vi "WS1021 demo GUI.vi"(6 "Error Limits file":path, 7 "VNA ports":bool[](array[boolean])=[TRUE, FALSE, FALSE, FALSE], 8 "Error In":errorcluster, 9 "De-embedding files":path[](array[path]), 10 "Toggle 8.lvclass":refnum<class "Toggle 8.lvclass">, 11 "Vector Network Analyzer.lvclass":refnum<class "Vector Network Analyzer.lvclass">) -> (0 "Error Out":errorcluster, 2 "Toggle 8.lvclass 2":refnum<class "Toggle 8.lvclass">, 3 "Vector Network Analyzer.lvclass 2":refnum<class "Vector Network Analyzer.lvclass">)   [LabVIEW 2020]
uses:
  Instruments/Vector Network Analyzer/Vector Network Analyzer.lvclass
  Devices/Toggle 8/Toggle 8.lvclass
  WS1021 demo GUI settings.ctl
  <vilib>/addons/HF Network Analysis/Support VIs/Read SnP File (SnP).vi
  <vilib>/addons/HF Network Analysis/NI_HFNetworkAnalysis.lvlib
  Devices/PIC-device/PIC-Device.lvclass
panel:
  out "Error limits":cluster{"Array":i32[], "Array":dbl[]}
  out "ErrorvsOTP":cluster{i32[], dbl[]}[](graph) caption="Capacitance error vs Setting"
  out "Heading":string[](array[string])=["Frequency (MHz)", "Capacitance (pF)", "Resistance (Ohm)", "Q", "Cshunt1 (pF)", "Cshunt2 (pF)", "SRF (MHz)"]
  out "Capacitance (pF) at f1":dbl caption="Capacitance (pF)\n at 900MHz" format="%#.2g"
  in  "Mode":enum32{"Automatic mode", "Manual mode"}(radio)
  in  "OTP":i32(slide)=1 caption="Capacitance setting" min=1 max=64 step=1 scale=1.0..64.0
  in  "Settings UI":bool
  in  "Pause Button":bool
  in  "Exit Button":bool
  out "Status bar":string
  out "Time":string
  in  "CvsOTP":cluster{"OTP":i32[], "Capa":dbl[]}
  out "Q at f2":dbl caption="Q-Value \nat 2000MHz" format="%#.1g"
  out "CvsOTP Graph":cluster{i32[], dbl[]}[](graph) caption="Capacitance vs Setting"
  in  "Demo Mode":enum32{"Live mode", "Virtual mode"}(radio)
  out "Capa Graph":cluster{dbl[], dbl[]}(graph) caption="Capacitance vs Frequency"
  out "Q Graph":cluster{dbl[], dbl[]}(graph) caption="Q vs Frequency"
  in  "Settings":T1={"Specification"={"States"=32, "Cmin"=250.0, "Cmax"=2600.0}, "Extraction frequencies"={"Frequency for C (MHz)"=900.0, "Frequency for Q (MHz)"=2000.0, "Frequency, C_DC (MHz)"=100.0}, "Timeout (ms)"=250, "Model"=enum."pi", "Topology"=enum."Series", "Error limits"=path ""}
  out "Status text box":string
  out "Data":dbl[][](array[numeric]) caption="Frequency,C, R, Q, L, Cshunt1/2, Rshunt1/2, Lshunt1/2, SRF"
  # "Digitally Tunable Capacitor"
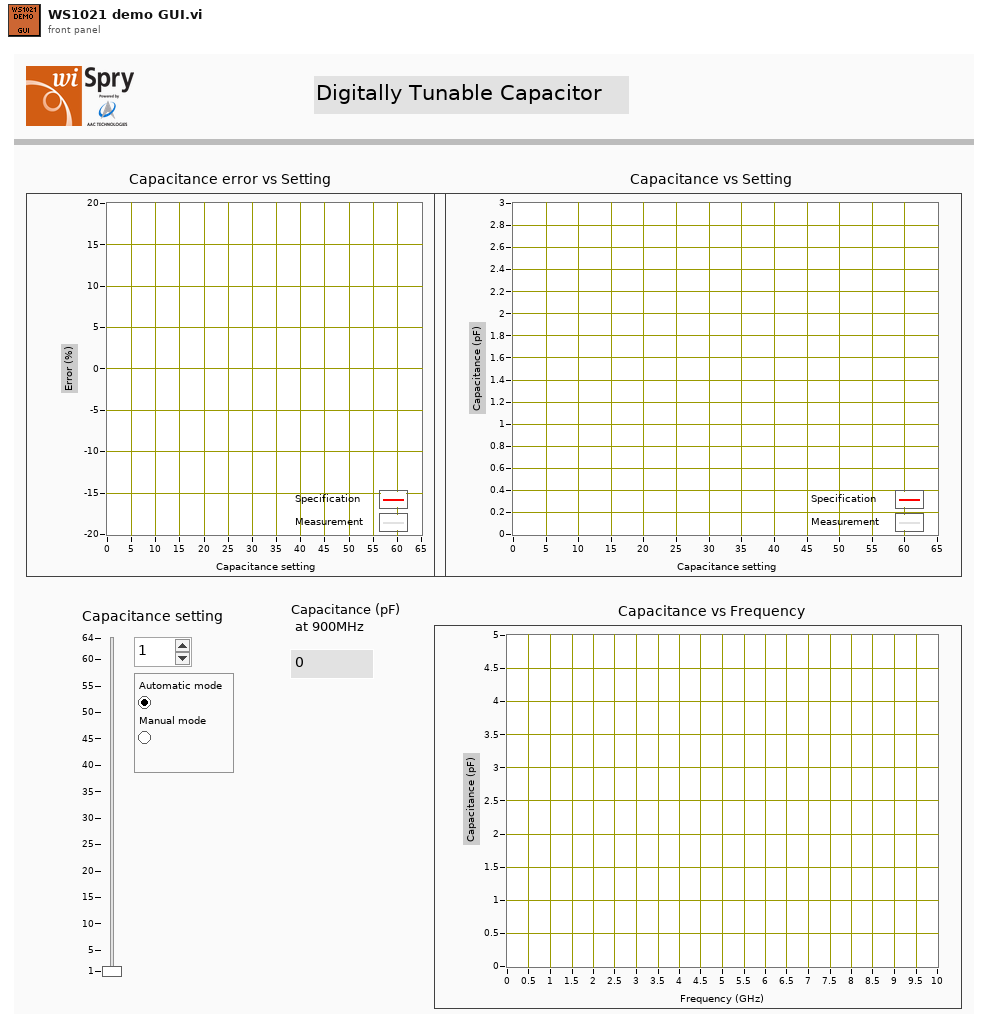
[diagram p1: front panel]
types:
  T1 = typedef "WS1021 demo GUI settings.ctl" = cluster{"Specification":cluster{"States":i32, "Cmin":dbl, "Cmax":dbl}, "Extraction frequencies":cluster{"Frequency for C (MHz)":dbl, "Frequency for Q (MHz)":dbl, "Frequency, C_DC (MHz)":dbl}, "Timeout (ms)":i32, "Model":enum16{"pi", "tee"}, "Topology":enum16{"Series", "Parallel"}, "Error limits":path}
  T2 = cluster{"Type":enum16{"Capacitor", "Switch"}, "Topology":enum16{"Series", "Parallel"}}
  T3 = enum8{"Enabled", "Disabled", "Disabled and Grayed Out"}
  T4 = typedef "Vector Network Analyzer.lvclass/Sparameter cluster.ctl" = cluster{"Frequency":dbl, "S Parameters":cdb[]}
  T5 = cluster{"Frequency for C (MHz)":dbl, "Frequency for Q (MHz)":dbl, "Frequency, C_DC (MHz)":dbl}
  T6 = cluster{cluster{"Frequencies (Hz) in":dbl[], dbl[]}, cluster{"Frequencies (Hz) in":dbl[], dbl[]}, cluster{"Frequencies (Hz) in":dbl[], dbl[]}[]}
  T7 = typedef "PIC-Device.lvclass/Register to Write.ctl" = cluster{"Register":u32, "Value":u32, "Dev Address":u32, "Physical Adress":u32}
  T8 = typedef "eventsource.ctl" = u32
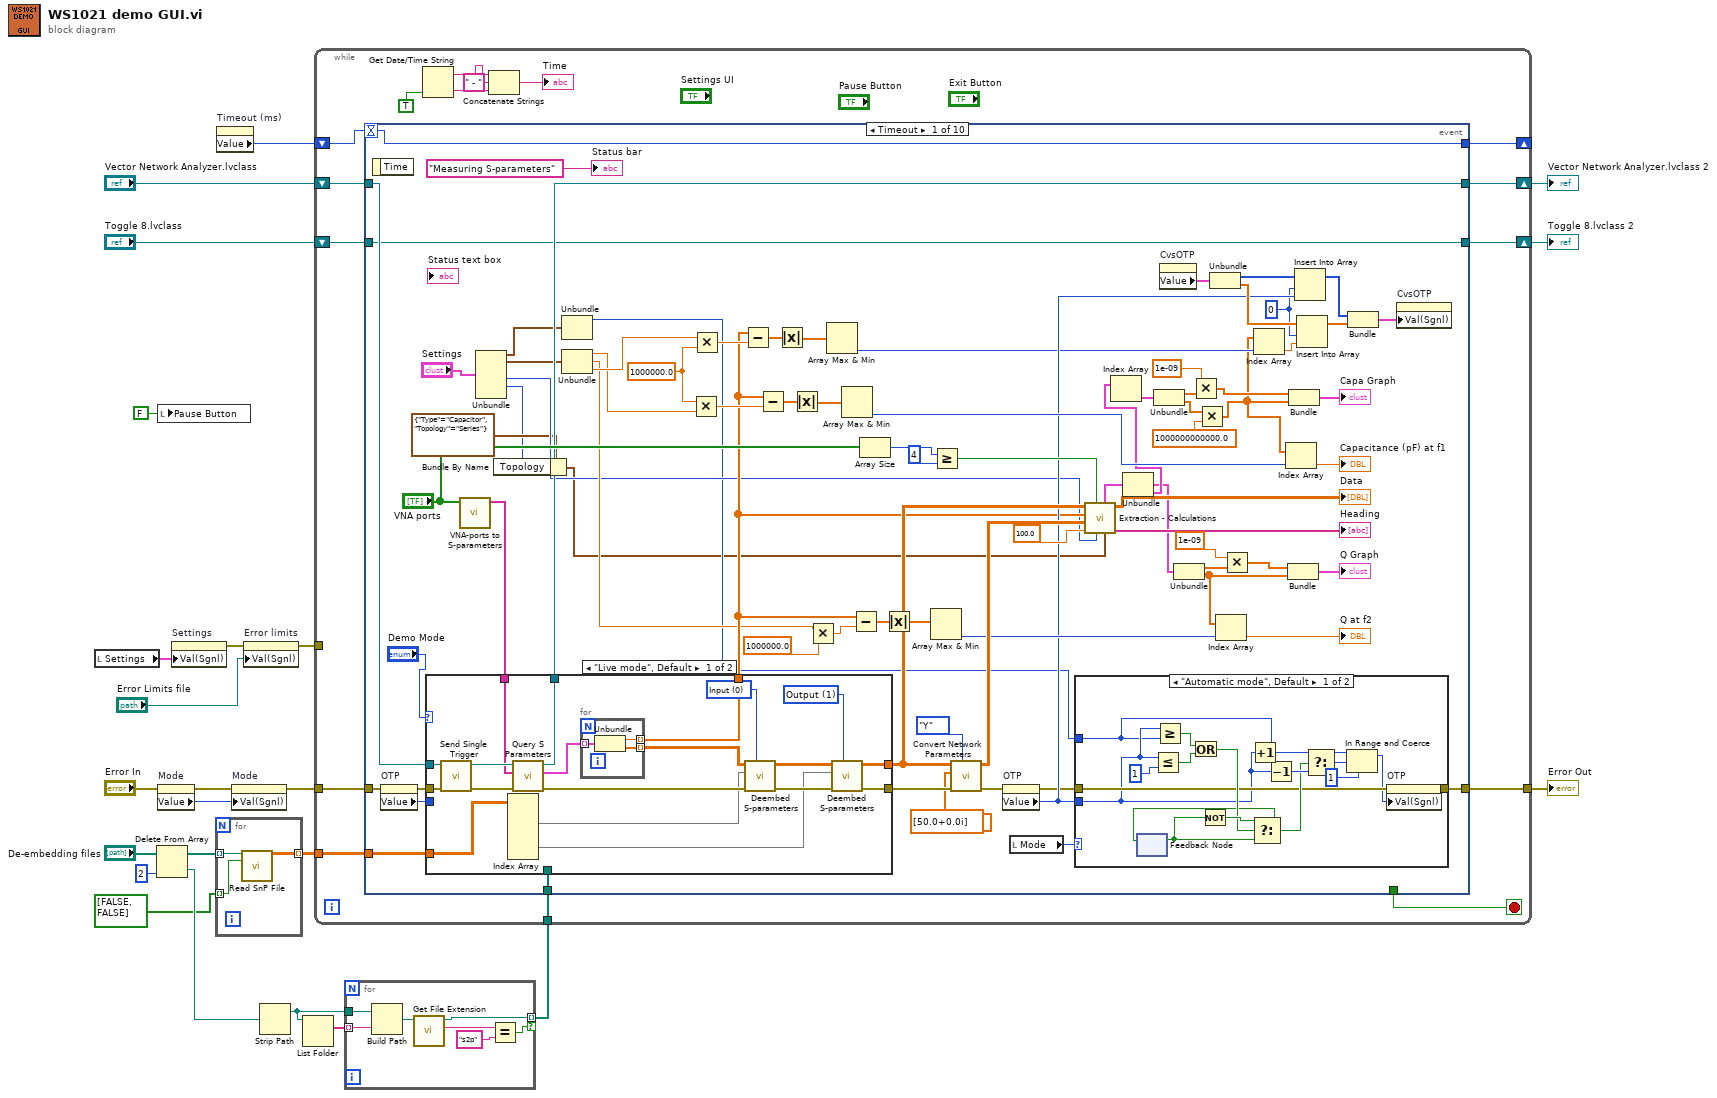
[diagram p0: block diagram]
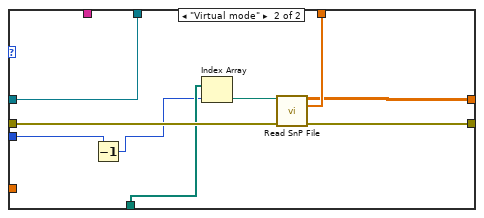
[diagram p2: hidden frame]
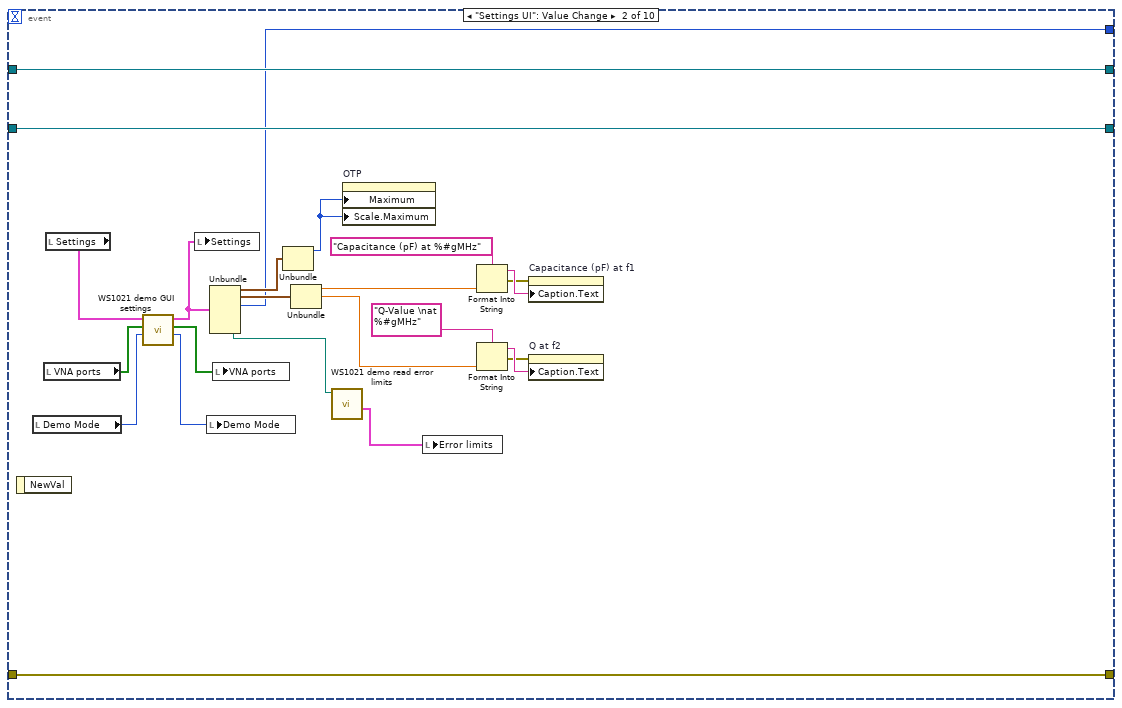
[diagram p4: hidden frame]
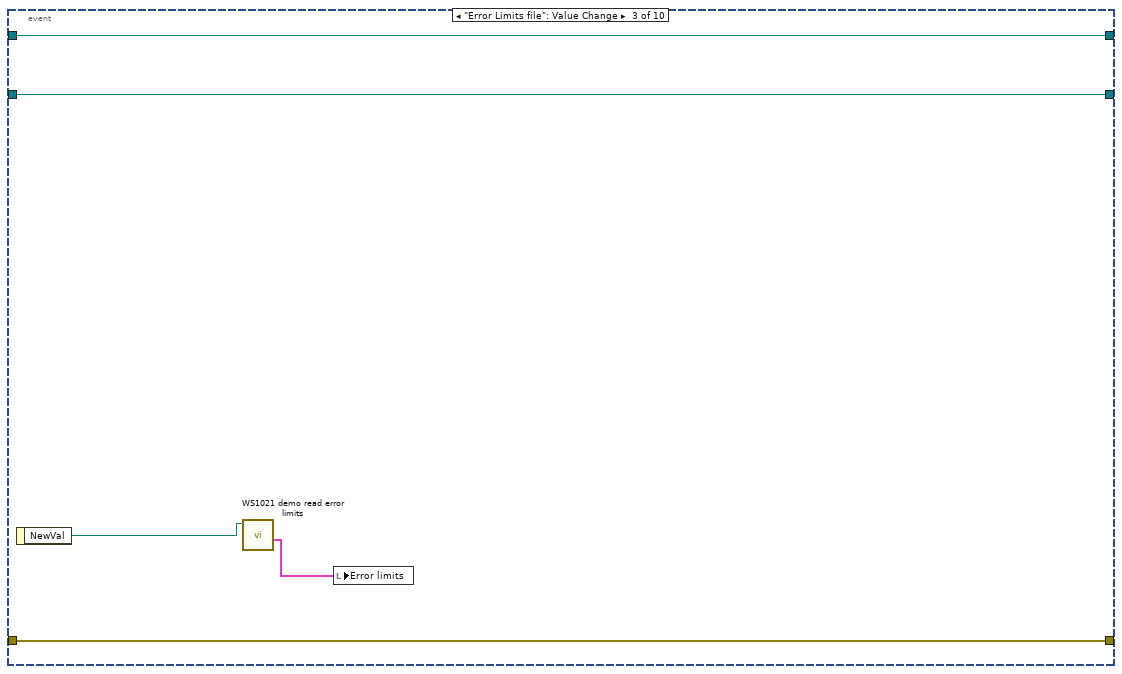
[diagram p5: hidden frame]
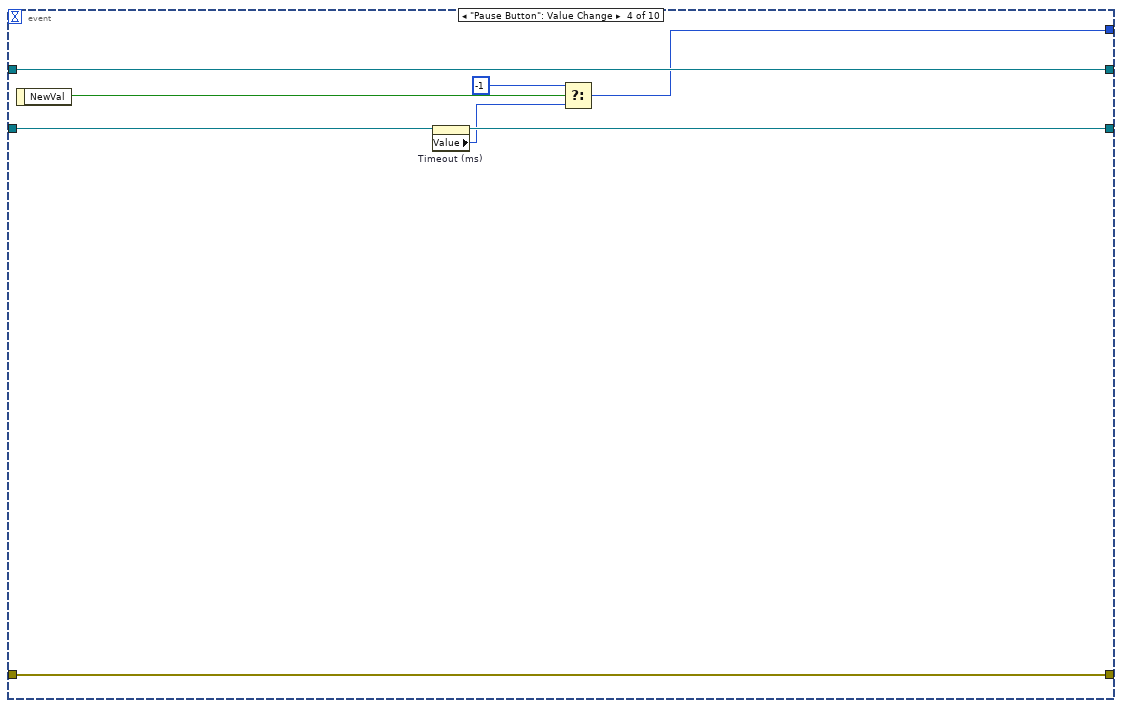
[diagram p6: hidden frame]
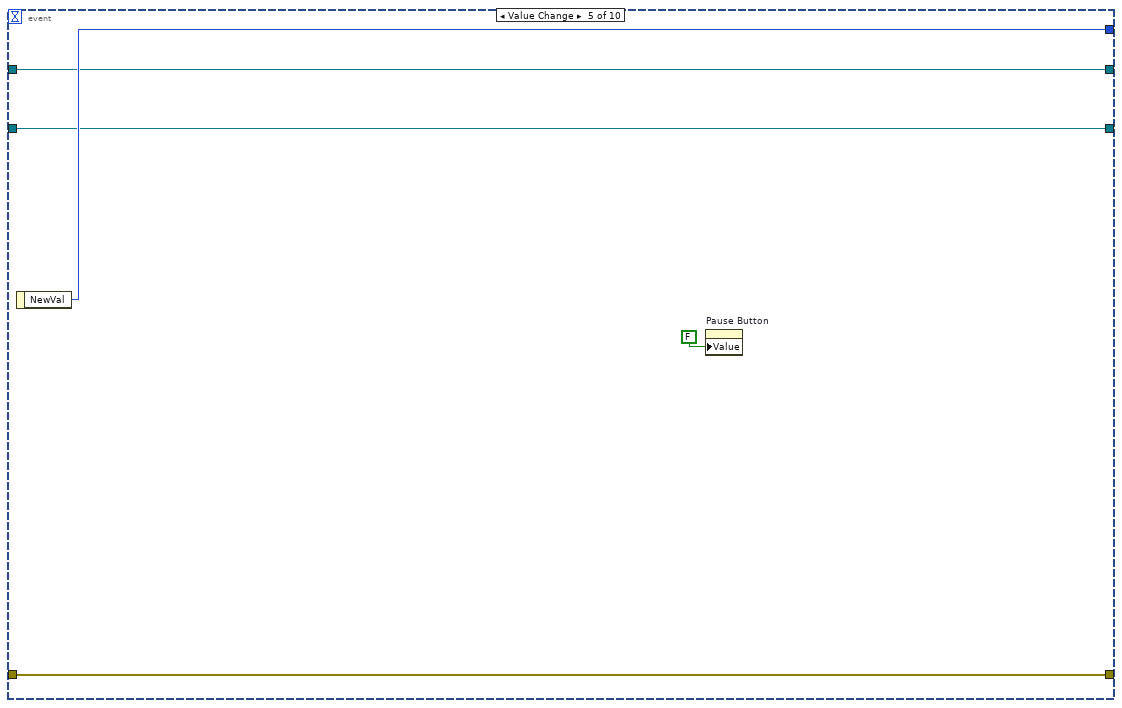
[diagram p7: hidden frame]
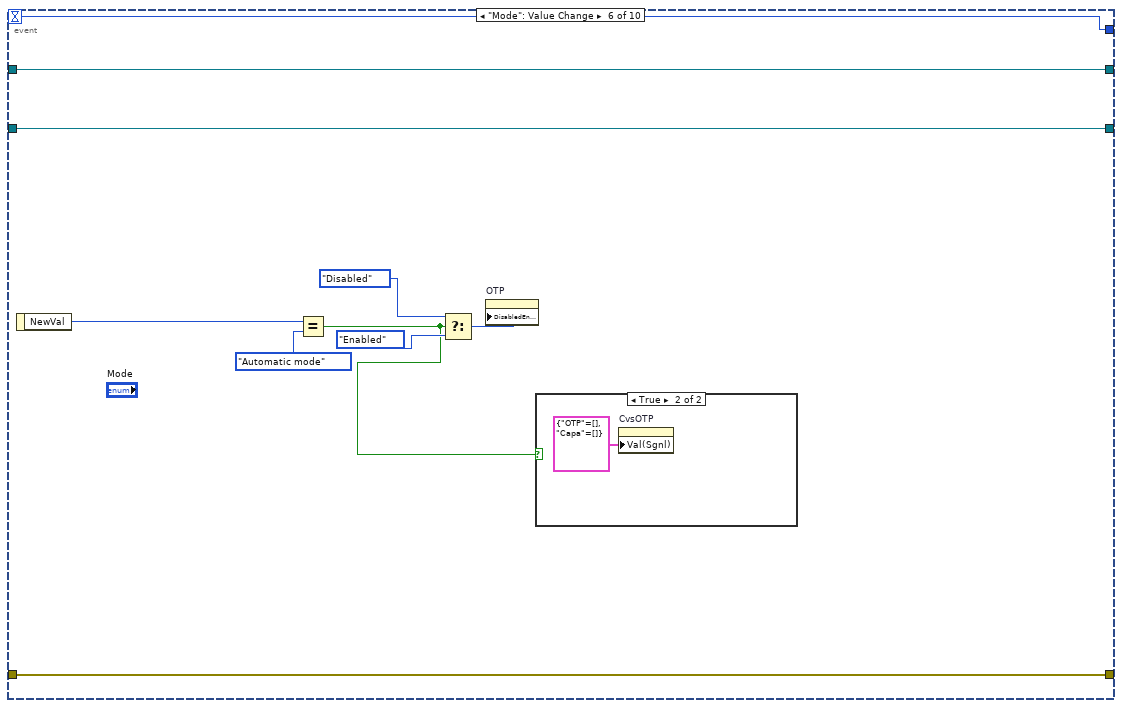
[diagram p8: hidden frame]
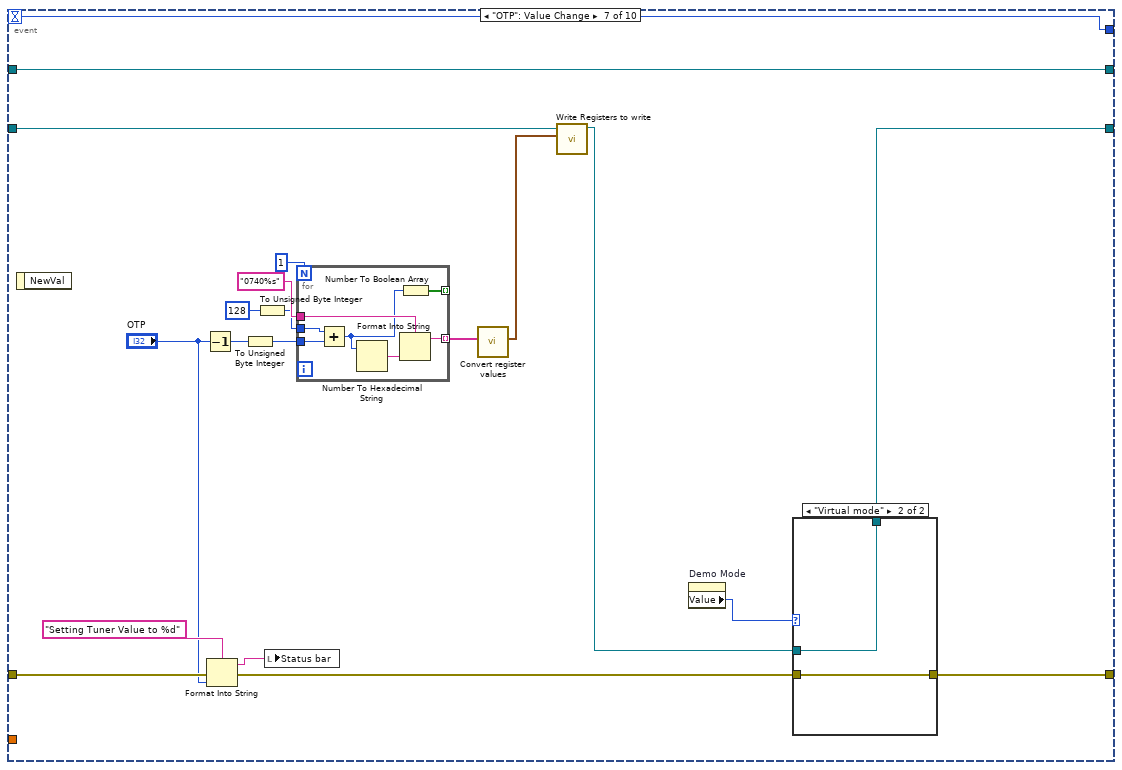
[diagram p10: hidden frame]
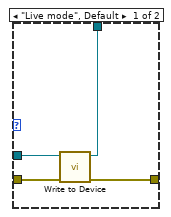
[diagram p11: hidden frame]
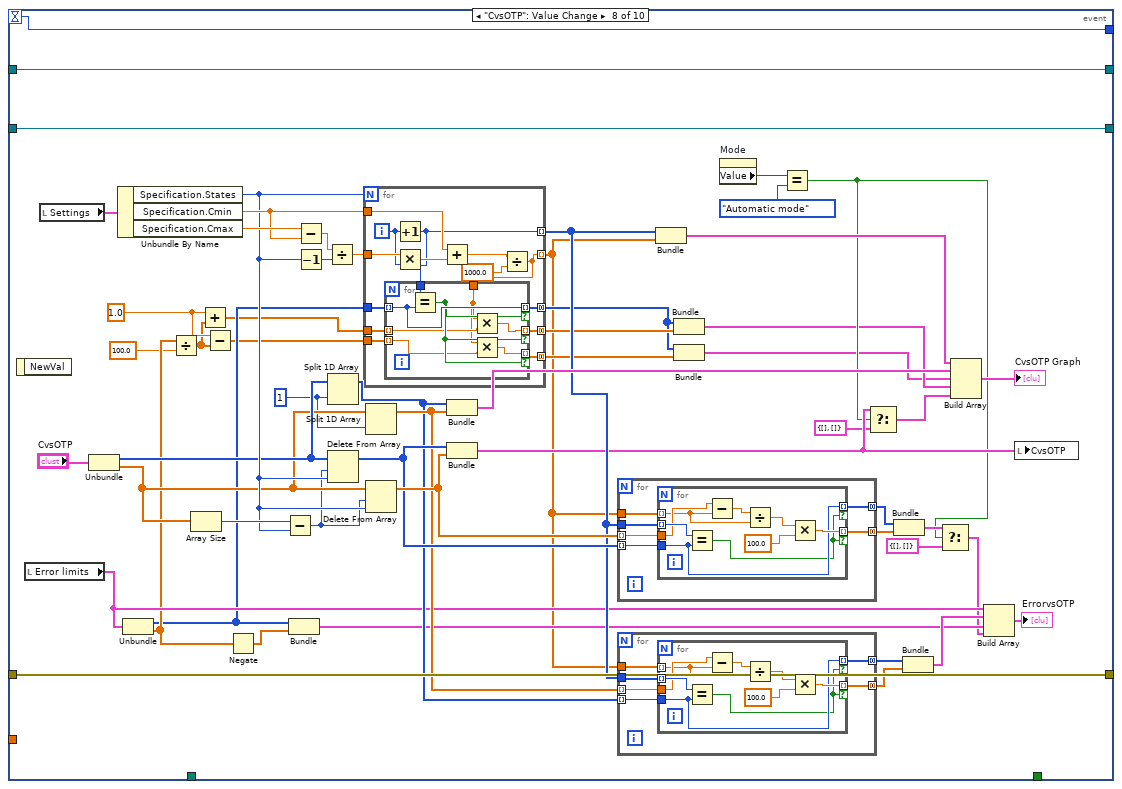
[diagram p12: hidden frame]
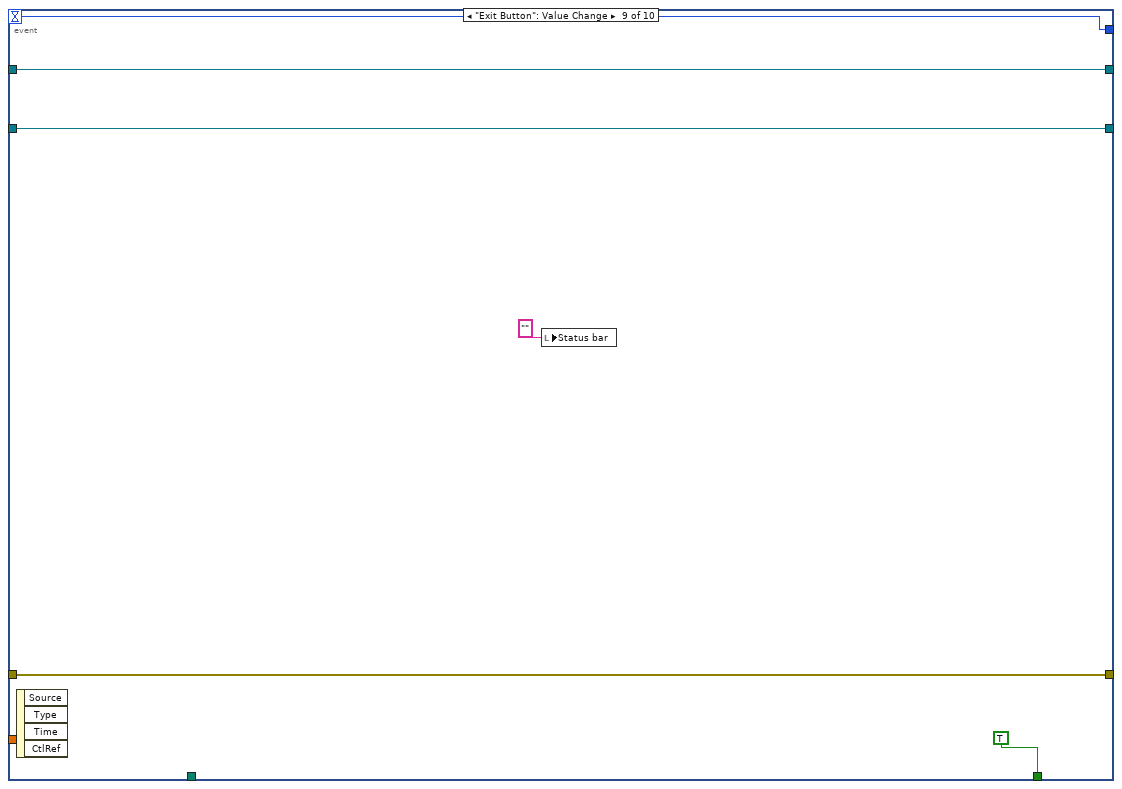
[diagram p13: hidden frame]
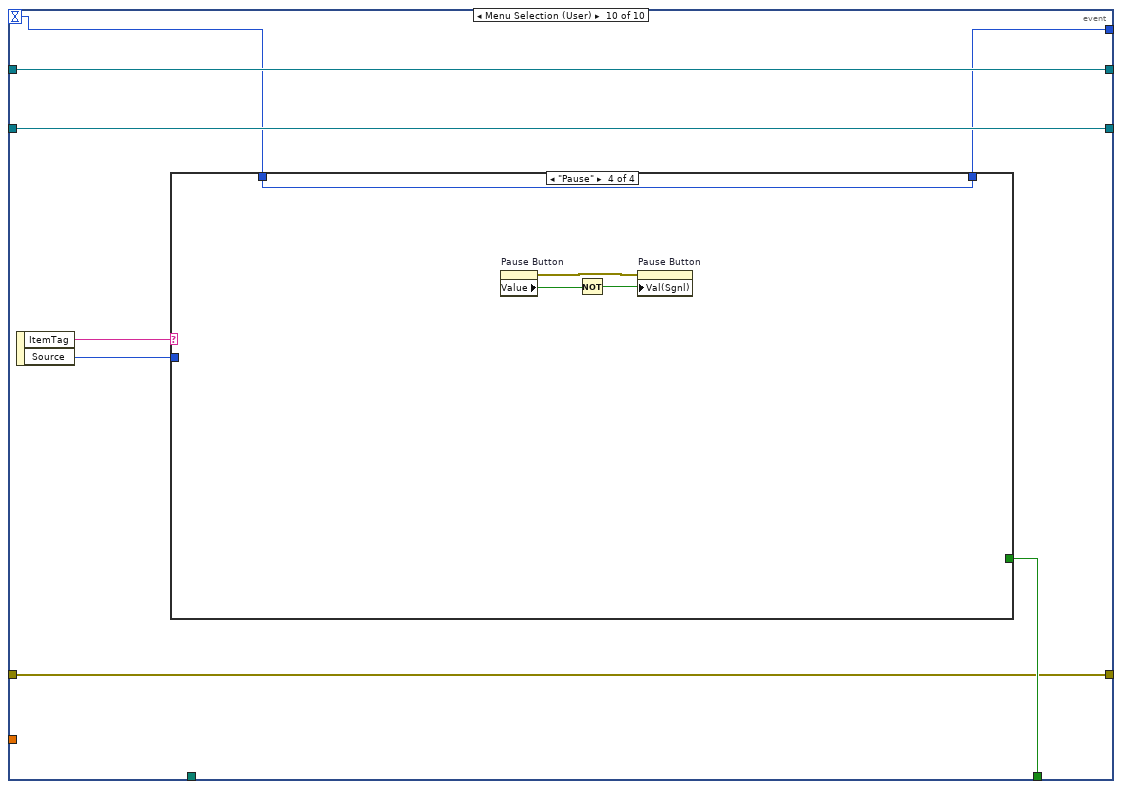
[diagram p14: hidden frame]
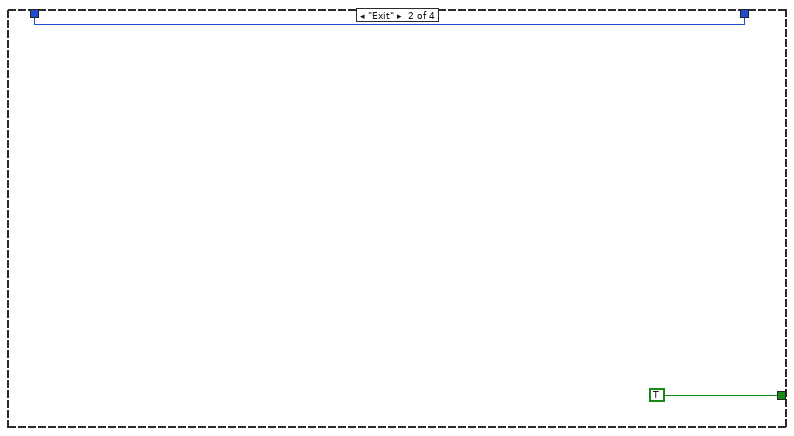
[diagram p16: hidden frame]
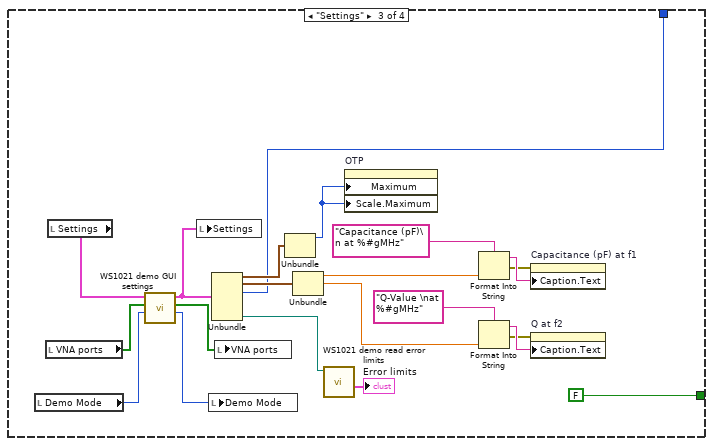
[diagram p17: hidden frame]
diagram:
  n1 = local read "Settings"() -> (w15:T1)
  n2 = Delete From Array(array="De-embedding files", index=2) -> (deleted portion=w6:path, array with subset deleted=w10:path[])  [unwired: 1 in]
  n3 = local write "Pause Button"(FALSE ("Pause Button")) -> ()
  n4 = property on="Mode" class="RadioBtnsControl (strict)"(error in="Error In") -> (error out=w23:errorcluster, "Value"=w24:enum32{"Automatic mode", "Manual mode"})  [unwired: 1 in, 1 out]
  n5 = property on="Settings" class="Clust (strict)"("Val(Sgnl)"=w15) -> (error out=w2:errorcluster)  [unwired: 2 in, 1 out]
  n6 = for {
    tunnel: w10 -> [w27] mode=indexing
    tunnel: [w26] -> w12 mode=indexing
    tunnel: bool[] [FALSE, FALSE] -> [w25] mode=indexing
    n7 = call-poly <vilib>:"Read SnP File.vi"("SnP File Path"=w27, "Swap Ports (False)"=w25) -> ("S-parameters"=w26:cdb[][])  [unwired: 10 in, 3 out]
  }
  n8 = property on="Timeout (ms)" class="DigNum (strict)"() -> ("Value"=w13:i32)  [unwired: 2 in, 2 out]
  n9 = property on="Mode" class="RadioBtnsControl (strict)"(error in=w23, "Val(Sgnl)"=w24) -> (error out=w21:errorcluster)  [unwired: 1 in, 1 out]
  n10 = property on="Error limits" class="Path"(error in=w2, "Val(Sgnl)"="Error Limits file") -> (error out=w1:errorcluster)  [unwired: 1 in, 1 out]
  n11 = Strip Path(path=w6) -> (stripped path=w8:path)  [unwired: 1 out]
  n12 = List Folder(path=w8) -> (filenames=w7:string[])  [unwired: 3 in, 3 out]
  n13 = for {
    tunnel: w8 -> [w31]
    tunnel: w7 -> [w30] mode=indexing
    tunnel: [w29] -> w5 mode=indexing if=w28
    n14 = Build Path(base path=w31, name or relative path=w30) -> (appended path=w32:path)
    n15 = call <vilib>:"Get File Extension.vi"("file"=w32) -> ("lowercase file extension"=w34:string, "dup file"=w29:path)  [unwired: 6 in, 3 out]
    n16 = Equal?(x=w34, y="s2p") -> (x = y?=w28:bool)
  }
  n17 = while {
    tunnel: w21 -> [w49]
    shift-right: [w45] -> w19
    shift-left: "Vector Network Analyzer.lvclass" -> [w48]
    tunnel: [w47] -> w18
    shift-right: [w44] -> w16
    shift-left: "Toggle 8.lvclass" -> [w46]
    shift-right: [w42] -> _
    shift-left: w13 -> [w43]
    tunnel: w12 -> [w36]
    tunnel: w5 -> [w35]
    tunnel: w1 -> [_]
    stop <- w50 stop-if-true
    n18 = event shown="[0] Timeout" {
      selector: _ -> [_ _ _ _ _ _ _ _ _ _]
      dyn-events: _ -> [_ _ _ _ _ _ _ _ _ _]
      timeout: w43 -> [w94 _ _ _ _ w221 w237 w317 w374 w380]
      tunnel: [_ _ _ _ _ _ _ _ TRUE w384] -> w50
      tunnel: w49 -> [w64 w196 w207 w212 w216 w222 w233 w310 w377 w383]
      tunnel: w48 -> [w124 w194 w203 w214 w218 w224 w250 w318 w376 w381]
      tunnel: [w118 w196 w207 w212 w216 w222 w240 w310 w377 w383] -> w47
      tunnel: w46 -> [w117 w195 w206 w213 w217 w223 w242 w319 w375 w382]
      tunnel: [w119 w194 w203 w214 w218 w224 w250 w318 w376 w381] -> w45
      tunnel: [w117 w195 w206 w213 w217 w223 w241 w319 w375 w382] -> w44
      tunnel: [w94 w184 _ w208 w219 w221 w237 w317 w374 w379] -> w42
      tunnel: w36 -> [w67 _ _ _ _ _ _ _ _ _]
      tunnel: w35 -> [w65 _ _ _ _ _ _ _ _ _]
      event Timeout {
        w79 = 0 ("index")
        w66 = 1000000.0 ("y")
        n19 = event-data() -> ()  [unwired: 1 in, 1 out]
        n20 = property on="OTP" class="Slide (strict)"(error in=w64) -> (error out=w63:errorcluster, "Value"=w62:i32)  [unwired: 1 in, 1 out]
        n21 = call "VNA-ports to S-parameters.vi"("VNA ports"="VNA ports") -> ("Sparameters (string)"=w131:string[])  [unwired: 6 in, 4 out]
        n22 = case shown="\"Live mode\", Default" "Demo Mode" {
          tunnel: w131 -> [w148 _]
          tunnel: w124 -> [w146 w162]
          tunnel: w63 -> [w145 w158]
          tunnel: [w142 w159] -> w121
          tunnel: [w137 w160] -> w120
          tunnel: [w136 w162] -> w119
          tunnel: [w135 w161] -> w80
          tunnel: w67 -> [w134 _]
          tunnel: w65 -> [_ w157]
          tunnel: w62 -> [_ w155]
          frame "Live mode", Default {
            w140 = u16 1 items=["Input", "Output"] ("Deembedding Side")
            w141 = u16 0 items=["Input", "Output"] ("Deembedding Side")
            n23 = call-dynamic "Send Single Trigger.vi"("error in (no error)"=w145, "Vector Network Analyzer in"=w146) -> ("error out"=w150:errorcluster, "Vector Network Analyzer out"=w149:refnum<class "Vector Network Analyzer.lvclass">)  [unwired: 8 in]
            n24 = Index Array(array=w134) -> (element #1=w133:cdb[][], element #2=w132:cdb[][])  [unwired: 6 in]
            n25 = call-dynamic "Query S Parameters.vi"("error in (no error)"=w150, "Sparameters (string)"=w148, "Vector Network Analyzer in"=w149) -> ("error out"=w144:errorcluster, "S parameters"=w147:T4[], "Vector Network Analyzer out"=w136:refnum<class "Vector Network Analyzer.lvclass">)  [unwired: 6 in]
            n26 = for {
              tunnel: w147 -> [w153] mode=indexing
              tunnel: [w152] -> w139 mode=indexing
              tunnel: [w151] -> w135 mode=indexing
              n27 = Unbundle(w153) -> ("Frequency"=w151:dbl, "S Parameters"=w152:cdb[])
            }
            n28 = call <vilib>:"Deembed S-parameters.vi"("Deembedding Side"=w141, "error in (no error)"=w144, "Deembedding S-par array in"=w133, "Original S-par array in"=w139) -> ("error out"=w143:errorcluster, "Deembedded S-par array out"=w138:cdb[][])  [unwired: 6 in]
            n29 = call <vilib>:"Deembed S-parameters.vi"("Deembedding Side"=w140, "error in (no error)"=w143, "Deembedding S-par array in"=w132, "Original S-par array in"=w138) -> ("error out"=w142:errorcluster, "Deembedded S-par array out"=w137:cdb[][])  [unwired: 6 in]
          }
          frame "Virtual mode" {
            n30 = Decrement(x=w155) -> (x-1=w154:i32)
            n31 = Index Array(array=w157, index=w154) -> (element=w156:path)
            n32 = call-poly <vilib>:"Read SnP File.vi"("SnP File Path"=w156, "Error In"=w158) -> ("S-parameters"=w160:cdb[][], "Frequencies (Hz)"=w161:dbl[], "Error Out"=w159:errorcluster)  [unwired: 10 in, 1 out]
          }
        }
        n33 = Unbundle("Settings") -> ("Specification"=w77:cluster{"States":i32, "Cmin":dbl, "Cmax":dbl}, "Extraction frequencies"=w76:T5, "Model"=w72:enum16{"pi", "tee"}, "Topology"=w56:enum16{"Series", "Parallel"})  [unwired: 2 out]
        n34 = Bundle By Name(cluster=T2 {"Type"=enum."Capacitor", "Topology"=enum."Series"} ("Device"), "Topology"=w56) -> (w55:T2)
        n35 = Unbundle(w77) -> ("States"=w71:i32)  [unwired: 2 out]
        n36 = Unbundle(w76) -> ("Frequency for C (MHz)"=w74:dbl, "Frequency for Q (MHz)"=w73:dbl, "Frequency, C_DC (MHz)"=w75:dbl)
        n37 = Multiply(x=w66, y=w74) -> (x*y=w108:dbl)
        n38 = Multiply(x=w75, y=w66) -> (x*y=w87:dbl)
        n39 = Subtract(x=w80, y=w87) -> (x-y=w89:dbl[])
        n40 = Subtract(x=w80, y=w108) -> (x-y=w115:dbl[])
        n41 = Absolute Value(x=w89) -> (abs(x)=w88:dbl[])
        n42 = Absolute Value(x=w115) -> (abs(x)=w113:dbl[])
        n43 = Multiply(x=w73, y=1000000.0) -> (x*y=w106:dbl)
        n44 = Array Max & Min(array=w88) -> (min index (indices)=w81:i32)  [unwired: 3 out]
        n45 = Array Max & Min(array=w113) -> (min index (indices)=w111:i32)  [unwired: 3 out]
        n46 = Subtract(x=w80, y=w106) -> (x-y=w114:dbl[])
        n47 = Array Size(array="VNA ports") -> (size(s)=w128:i32)
        n48 = Absolute Value(x=w114) -> (abs(x)=w112:dbl[])
        n49 = Array Max & Min(array=w112) -> (min index (indices)=w109:i32)  [unwired: 3 out]
        n50 = Greater Or Equal?(x=w128, y=4) -> (x >= y?=w126:bool)
        n51 = call "Convert Network Parameters.vi"("Parameters to convert"=enum16{"Y", "Z", "T"}."Y", "error in (no error)"=w121, "Zc (Ohm)"=cdb[] [50.0+0.0i], "S-par Array In"=w120) -> ("error out"=w61:errorcluster, "Y/Z Array Out"=w130:cdb[][])  [unwired: 5 in, 1 out]
        n52 = property on="OTP" class="Slide (strict)"(error in=w61) -> (error out=w60:errorcluster, "Value"=w90:i32)  [unwired: 1 in, 1 out]
        n53 = local read "Mode"() -> (w116:enum32{"Automatic mode", "Manual mode"})
        n54 = case shown="\"Automatic mode\", Default" w116 {
          tunnel: w60 -> [w168 w179]
          tunnel: [w176 w179] -> w118
          tunnel: w90 -> [w167 _]
          tunnel: w71 -> [w163 _]
          frame "Automatic mode", Default {
            n55 = feedback #1() -> (w174:bool)  [unwired: 1 in]
            n56 = Less Or Equal?(x=w167, y=1) -> (x <= y?=w171:bool)
            n57 = Greater Or Equal?(x=w167, y=w163) -> (x >= y?=w172:bool)
            n58 = Or(x=w172, y=w171) -> (x .or. y?=w170:bool)
            n59 = Not(x=w174) -> (.not. x?=w175:bool)
            n60 = Increment(x=w167) -> (x+1=w177:i32)
            n61 = Select(t=w175, s=w170, f=w174) -> (s? t:f=w169:bool)
            n62 = feedback-in #1(w169) -> ()
            n63 = Decrement(x=w167) -> (x-1=w178:i32)
            n64 = Select(t=w177, s=w169, f=w178) -> (s? t:f=w165:i32)
            n65 = In Range and Coerce(upper limit=w163, x=w165, lower limit=1) -> (coerced(x)=w164:i32)  [unwired: 1 out]
            n66 = property on="OTP" class="Slide (strict)"(error in=w168, "Val(Sgnl)"=w164) -> (error out=w176:errorcluster)  [unwired: 1 in, 1 out]
          }
          frame "Manual mode" {
          }
        }
        n67 = call "Extraction - Calculations.vi"("Device"=w55, "Model"=w72, "2-port?"=w126, "Freq for nominal C (MHz)"=100.0, "Y/Z-parameters"=w130, "Frequencies (Hz) in"=w80, "S-parameters"=w120) -> ("Heading"=→"Heading":string[], "Frequency,C, R, Q/-IL, L, Cshunt1/2, Rshunt1/2, Lshunt1/2, SRF"=→"Data":dbl[][], "Graphs"=w53:T6)  [unwired: 2 out]
        n68 = Unbundle(w53) -> (w51:cluster{"Frequencies (Hz) in":dbl[], dbl[]}, w52:cluster{"Frequencies (Hz) in":dbl[], dbl[]}[])  [unwired: 1 out]
        n69 = Index Array(array=w52) -> (element=w98:cluster{"Frequencies (Hz) in":dbl[], dbl[]})  [unwired: 1 in]
        n70 = Unbundle(w98) -> ("Frequencies (Hz) in"=w96:dbl[], w59:dbl[])
        n71 = property on="CvsOTP" class="Clust (strict)"() -> ("Value"=w93:cluster{"OTP":i32[], "Capa":dbl[]})  [unwired: 2 in, 2 out]
        n72 = Unbundle(w51) -> ("Frequencies (Hz) in"=w102:dbl[], w101:dbl[])
        n73 = Multiply(x=1e-09 ("y"), y=w96) -> (x*y=w95:dbl[])
        n74 = Multiply(x=w59, y=1000000000000.0) -> (x*y=w58:dbl[])
        n75 = Unbundle(w93) -> ("OTP"=w92:i32[], "Capa"=w91:dbl[])
        n76 = Index Array(array=w101, index=w109) -> (element=→"Q at f2":dbl)
        n77 = Multiply(x=1e-09 ("y"), y=w102) -> (x*y=w103:dbl[])
        n78 = Index Array(array=w58, index=w81) -> (element=w83:dbl)
        n79 = Index Array(array=w58, index=w111) -> (element=→"Capacitance (pF) at f1":dbl)
        n80 = Bundle(w103, w101) -> (→"Q Graph":cluster{dbl[], dbl[]})  [unwired: 1 in]
        n81 = Bundle(w95, w58) -> (→"Capa Graph":cluster{dbl[], dbl[]})  [unwired: 1 in]
        n82 = Insert Into Array(array=w92, index=w79, new element=w90) -> (w85:i32[])
        n83 = Insert Into Array(array=w91, index=w79, new element=w83) -> (w86:dbl[])
        n84 = Bundle("OTP"=w85, "Capa"=w86) -> (w84:cluster{"OTP":i32[], "Capa":dbl[]})  [unwired: 1 in]
        n85 = property on="CvsOTP" class="Clust (strict)"("Val(Sgnl)"=w84) -> ()  [unwired: 2 in, 2 out]
        "Status bar" <- "Measuring S-parameters" ("Status bar")
      }
      event "Settings UI": Value Change {
        n86 = event-data() -> ()  [unwired: 1 in, 1 out]
        n87 = local read "Demo Mode"() -> (w183:enum32{"Live mode", "Virtual mode"})
        n88 = local read "VNA ports"() -> (w187:bool[])
        n89 = local read "Settings"() -> (w188:T1)
        n90 = call "WS1021 demo GUI settings.vi"("Demo Mode"=w183, "VNA ports"=w187, "Settings"=w188) -> ("Demo Mode out"=w182:enum32{"Live mode", "Virtual mode"}, "VNA ports out"=w186:bool[], "Settings out"=w185:T1)  [unwired: 6 in]
        n91 = local write "Settings"(w185) -> ()
        n92 = local write "Demo Mode"(w182) -> ()
        n93 = Unbundle(w185) -> ("Specification"=w193:cluster{"States":i32, "Cmin":dbl, "Cmax":dbl}, "Extraction frequencies"=w192:T5, "Timeout (ms)"=w184:i32, "Error limits"=w181:path)  [unwired: 2 out]
        n94 = local write "VNA ports"(w186) -> ()
        n95 = Unbundle(w193) -> ("States"=w189:i32)  [unwired: 2 out]
        n96 = Unbundle(w192) -> ("Frequency for C (MHz)"=w191:dbl, "Frequency for Q (MHz)"=w190:dbl)  [unwired: 1 out]
        n97 = call "WS1021 demo read error limits.vi"("file path (dialog if empty)"=w181) -> ("Error limits"=w180:cluster{"Array":i32[], "Array":dbl[]})  [unwired: 8 in, 2 out]
        n98 = property on="OTP" class="Slide (strict)"("Maximum"=w189, "Scale.Maximum"=w189) -> ()  [unwired: 2 in, 2 out]
        n99 = local write "Error limits"(w180) -> ()
        n100 = Format Into String(format string="Capacitance (pF) at %#gMHz", w191) -> (resulting string=w199:string, error out=w198:errorcluster)  [unwired: 2 in]
        n101 = Format Into String(format string="Q-Value \nat %#gMHz", w190) -> (resulting string=w200:string, error out=w197:errorcluster)  [unwired: 2 in]
        n102 = property on="Capacitance (pF) at f1" class="DigNum (strict)"(error in=w198, "Caption.Text"=w199) -> ()  [unwired: 1 in, 2 out]
        n103 = property on="Q at f2" class="DigNum (strict)"(error in=w197, "Caption.Text"=w200) -> ()  [unwired: 1 in, 2 out]
      }
      event "Error Limits file": Value Change {
        n104 = event-data() -> ("NewVal"=w204:path)  [unwired: 1 in]
        n105 = call "WS1021 demo read error limits.vi"("file path (dialog if empty)"=w204) -> ("Error limits"=w205:cluster{"Array":i32[], "Array":dbl[]})  [unwired: 8 in, 2 out]
        n106 = local write "Error limits"(w205) -> ()
      }
      event "Pause Button": Value Change {
        n107 = event-data() -> ("NewVal"=w211:bool)  [unwired: 1 in]
        n108 = property on="Timeout (ms)" class="DigNum (strict)"() -> ("Value"=w210:i32)  [unwired: 2 in, 2 out]
        n109 = Select(t=-1, s=w211, f=w210) -> (s? t:f=w208:i32)
      }
      event Value Change {
        n110 = event-data() -> ("NewVal"=w219:i32)  [unwired: 1 in]
        n111 = property on="Pause Button" class="Bool (strict)"("Value"=FALSE ("Pause Button")) -> ()  [unwired: 2 in, 2 out]
      }
      event "Mode": Value Change {
        n112 = event-data() -> ("NewVal"=w229:enum32{"Automatic mode", "Manual mode"})  [unwired: 1 in]
        n113 = Equal?(x=w229, y=enum32{"Automatic mode", "Manual mode"}."Automatic mode") -> (x = y?=w220:bool)
        n114 = Select(t=T3."Disabled" ("Disabled"), s=w220, f=T3."Enabled" ("Disabled")) -> (s? t:f=w225:T3)
        n115 = property on="OTP" class="Slide (strict)"("DisabledEnum"=w225) -> ()  [unwired: 2 in, 2 out]
        n116 = case shown="True" w220 {
          frame False {
          }
          frame True {
            n117 = property on="CvsOTP" class="Clust (strict)"("Val(Sgnl)"=cluster{"OTP":i32[], "Capa":dbl[]} {"OTP"=[], "Capa"=[]} ("Value (Signaling)")) -> ()  [unwired: 2 in, 2 out]
          }
        }
      }
      event "OTP": Value Change {
        n118 = event-data() -> ()  [unwired: 1 in, 1 out]
        n119 = Decrement(x="OTP") -> (x-1=w238:i32)
        n120 = Format Into String(format string="Setting Tuner Value to %d" ("Status bar"), error in=w233, "OTP") -> (resulting string=w235:string, error out=w234:errorcluster)  [unwired: 1 in]
        n121 = To Unsigned Byte Integer(number=w238) -> (unsigned 8bit integer=w247:u8)
        n122 = To Unsigned Byte Integer(number=u8 128) -> (unsigned 8bit integer=w245:u8)
        n123 = local write "Status bar"(w235) -> ()
        n124 = for {
          N: 1 -> [_]
          tunnel: w247 -> [w259]
          tunnel: "0740%s" -> [w263]
          tunnel: [w262] -> _ mode=indexing
          tunnel: w245 -> [w261]
          tunnel: [w257] -> w244 mode=indexing
          n125 = Add(x=w261, y=w259) -> (x+y=w260:u8)
          n126 = Number To Hexadecimal String(2:w260) -> (0:w258:string)  [unwired: 1 in]
          n127 = Format Into String(format string=w263, w258) -> (resulting string=w257:string)  [unwired: 2 in, 1 out]
          n128 = Number To Boolean Array(number=w260) -> (Boolean array=w262:bool[])
        }
        n129 = call "Convert register values.vi"("Register strings"=w244) -> ("Register clusters out"=w243:T7[])  [unwired: 9 in, 1 out]
        n130 = call-dynamic "Write Registers to write.vi"("Registers to write"=w243, "Device in"=w242) -> ("Device out"=w249:refnum<class "Toggle 8.lvclass">)  [unwired: 9 in]
        n131 = property on="Demo Mode" class="RadioBtnsControl (strict)"() -> ("Value"=w231:enum32{"Live mode", "Virtual mode"})  [unwired: 2 in, 2 out]
        n132 = case shown="\"Virtual mode\"" w231 {
          tunnel: w249 -> [w254 w255]
          tunnel: [w253 w255] -> w241
          tunnel: [w252 w256] -> w240
          tunnel: w234 -> [w251 w256]
          frame "Live mode", Default {
            n133 = call-dynamic "Write to Device.vi"("error in (no error)"=w251, "Device in"=w254) -> ("error out"=w252:errorcluster, "Device out"=w253:refnum<class "Toggle 8.lvclass">)  [unwired: 7 in, 1 out]
          }
          frame "Virtual mode" {
          }
        }
      }
      event "CvsOTP": Value Change {
        w274 = 1.0
        w295 = 1
        n134 = event-data() -> ()  [unwired: 1 in, 1 out]
        n135 = local read "Error limits"() -> (w287:cluster{"Array":i32[], "Array":dbl[]})
        n136 = local read "Settings"() -> (w309:T1)
        n137 = Unbundle("CvsOTP") -> ("OTP"=w299:i32[], "Capa"=w298:dbl[])
        n138 = Unbundle By Name(w309) -> ("Specification.States"=w300:i32, "Specification.Cmin"=w307:dbl, "Specification.Cmax"=w308:dbl)
        n139 = Unbundle(w287) -> ("Array"=w270:i32[], "Array"=w276:dbl[])
        n140 = Divide(x=w276, y=100.0) -> (x/y=w273:dbl[])
        n141 = Array Size(array=w298) -> (size(s)=w306:i32)
        n142 = Add(x=w274, y=w273) -> (x+y=w269:dbl[])
        n143 = Subtract(x=w274, y=w273) -> (x-y=w268:dbl[])
        n144 = Negate(x=w276) -> (-x=w288:dbl[])
        n145 = Subtract(x=w306, y=w300) -> (x-y=w297:i32)
        n146 = Bundle("Array"=w270, w288) -> (w286:cluster{"Array":i32[], dbl[]})  [unwired: 1 in]
        n147 = Subtract(x=w308, y=w307) -> (x-y=w316:dbl)
        n148 = Decrement(x=w300) -> (x-1=w314:i32)
        n149 = Divide(x=w316, y=w314) -> (x/y=w315:dbl)
        n150 = Split 1D Array(array=w299, index=w295) -> (first subarray=w292:i32[])  [unwired: 1 out]
        n151 = Delete From Array(array=w299, length=w297, index=w300) -> (array with subset deleted=w303:i32[])  [unwired: 1 out]
        n152 = for {
          N: w300 -> [_]
          tunnel: w315 -> [w363]
          tunnel: [w350] -> w264 mode=indexing
          tunnel: [w359] -> w294 mode=indexing
          tunnel: w307 -> [w361]
          tunnel: w270 -> [w358]
          tunnel: w269 -> [w357]
          tunnel: w268 -> [w356]
          tunnel: [w355] -> w267 mode=concatenating
          tunnel: [w354] -> w266 mode=concatenating
          tunnel: [w353] -> w265 mode=concatenating
          i -> [w362]
          n153 = Increment(x=w362) -> (x+1=w359:i32)
          n154 = Multiply(x=w363, y=w362) -> (x*y=w360:dbl)
          n155 = Add(x=w361, y=w360) -> (x+y=w351:dbl)
          n156 = Divide(x=w351, y=1000.0) -> (x/y=w350:dbl)
          n157 = for {
            tunnel: w359 -> [w371]
            tunnel: w358 -> [w370] mode=indexing
            tunnel: w357 -> [w367] mode=indexing
            tunnel: w356 -> [w368] mode=indexing
            tunnel: [w364] -> w355 mode=indexing if=w369
            tunnel: [w365] -> w354 mode=indexing if=w369
            tunnel: [w370] -> w353 mode=indexing if=w369
            tunnel: w350 -> [w366]
            n158 = Equal?(x=w371, y=w370) -> (x = y?=w369:bool)
            n159 = Multiply(x=w366, y=w367) -> (x*y=w364:dbl)
            n160 = Multiply(x=w366, y=w368) -> (x*y=w365:dbl)
          }
        }
        n161 = Split 1D Array(array=w298, index=w295) -> (first subarray=w293:dbl[])  [unwired: 1 out]
        n162 = Delete From Array(array=w298, length=w297, index=w300) -> (array with subset deleted=w304:dbl[])  [unwired: 1 out]
        n163 = Bundle(w292, w293) -> (w296:cluster{i32[], dbl[]})  [unwired: 1 in]
        n164 = Bundle("OTP"=w303, "Capa"=w304) -> (w282:cluster{"OTP":i32[], "Capa":dbl[]})  [unwired: 1 in]
        n165 = for {
          tunnel: w303 -> [w339] mode=indexing
          tunnel: w294 -> [w340]
          tunnel: w264 -> [w338]
          tunnel: w304 -> [w337] mode=indexing
          tunnel: [w336] -> w301 mode=concatenating
          tunnel: [w335] -> w302 mode=concatenating
          n166 = for {
            tunnel: w340 -> [w349] mode=indexing
            tunnel: w339 -> [w342]
            tunnel: w338 -> [w344] mode=indexing
            tunnel: w337 -> [w345]
            tunnel: [w343] -> w336 mode=indexing if=w341
            tunnel: [w342] -> w335 mode=indexing if=w341
            n167 = Equal?(x=w349, y=w342) -> (x = y?=w341:bool)
            n168 = Subtract(x=w345, y=w344) -> (x-y=w348:dbl)
            n169 = Divide(x=w348, y=w344) -> (x/y=w347:dbl)
            n170 = Multiply(x=w347, y=100.0) -> (x*y=w343:dbl)
          }
        }
        n171 = for {
          tunnel: w292 -> [w324] mode=indexing
          tunnel: w294 -> [w325]
          tunnel: w264 -> [w323]
          tunnel: w293 -> [w322] mode=indexing
          tunnel: [w321] -> w290 mode=concatenating
          tunnel: [w320] -> w291 mode=concatenating
          n172 = for {
            tunnel: w325 -> [w334] mode=indexing
            tunnel: w324 -> [w327]
            tunnel: w323 -> [w329] mode=indexing
            tunnel: w322 -> [w330]
            tunnel: [w328] -> w321 mode=indexing if=w326
            tunnel: [w327] -> w320 mode=indexing if=w326
            n173 = Equal?(x=w334, y=w327) -> (x = y?=w326:bool)
            n174 = Subtract(x=w330, y=w329) -> (x-y=w333:dbl)
            n175 = Divide(x=w333, y=w329) -> (x/y=w332:dbl)
            n176 = Multiply(x=w332, y=100.0) -> (x*y=w328:dbl)
          }
        }
        n177 = Bundle(w294, w264) -> (w312:cluster{i32[], dbl[]})  [unwired: 1 in]
        n178 = Bundle(w265, w267) -> (w272:cluster{i32[], dbl[]})  [unwired: 1 in]
        n179 = Bundle(w265, w266) -> (w271:cluster{i32[], dbl[]})  [unwired: 1 in]
        n180 = property on="Mode" class="RadioBtnsControl (strict)"() -> ("Value"=w285:enum32{"Automatic mode", "Manual mode"})  [unwired: 2 in, 2 out]
        n181 = Equal?(x=w285, y=enum32{"Automatic mode", "Manual mode"}."Automatic mode") -> (x = y?=w277:bool)
        n182 = Select(t=w282, s=w277, f=cluster{i32[], dbl[]} {[], []} ("cluster")) -> (s? t:f=w283:cluster{"OTP":i32[], "Capa":dbl[]})
        n183 = Bundle(w302, w301) -> (w279:cluster{i32[], dbl[]})  [unwired: 1 in]
        n184 = Bundle(w291, w290) -> (w289:cluster{i32[], dbl[]})  [unwired: 1 in]
        n185 = Select(t=w279, s=w277, f=cluster{i32[], dbl[]} {[], []} ("cluster")) -> (s? t:f=w278:cluster{i32[], dbl[]})
        n186 = Build Array(w312, w296, w271, w272, w283) -> (→"CvsOTP Graph":cluster{"OTP":i32[], "Capa":dbl[]}[])
        n187 = Build Array(w287, w289, w286, w278) -> (→"ErrorvsOTP":cluster{"Array":i32[], "Array":dbl[]}[])
        n188 = local write "CvsOTP"(w282) -> ()
      }
      event "Exit Button": Value Change {
        n189 = event-data() -> ()  [unwired: 1 in, 4 out]
        n190 = local write "Status bar"("" ("Status bar")) -> ()
      }
      event Menu Selection (User) {
        n191 = event-data() -> ("ItemTag"=w385:string, "Source"=w378:T8)  [unwired: 1 in]
        n192 = case shown="\"Pause\"" w385 {
          tunnel: [_ TRUE FALSE _] -> w384
          tunnel: [w386 w387 w391 w410] -> w379
          tunnel: w380 -> [w386 w387 _ w410]
          tunnel: w378 -> [_ _ _ _]
          frame Default {
          }
          frame "Exit" {
          }
          frame "Settings" {
            n193 = local read "Demo Mode"() -> (w395:enum32{"Live mode", "Virtual mode"})
            n194 = local read "VNA ports"() -> (w398:bool[])
            n195 = local read "Settings"() -> (w399:T1)
            n196 = call "WS1021 demo GUI settings.vi"("Demo Mode"=w395, "VNA ports"=w398, "Settings"=w399) -> ("Demo Mode out"=w394:enum32{"Live mode", "Virtual mode"}, "VNA ports out"=w397:bool[], "Settings out"=w396:T1)  [unwired: 6 in]
            n197 = local write "Settings"(w396) -> ()
            n198 = local write "Demo Mode"(w394) -> ()
            n199 = Unbundle(w396) -> ("Specification"=w404:cluster{"States":i32, "Cmin":dbl, "Cmax":dbl}, "Extraction frequencies"=w403:T5, "Timeout (ms)"=w391:i32, "Error limits"=w390:path)  [unwired: 2 out]
            n200 = local write "VNA ports"(w397) -> ()
            n201 = Unbundle(w404) -> ("States"=w400:i32)  [unwired: 2 out]
            n202 = Unbundle(w403) -> ("Frequency for C (MHz)"=w402:dbl, "Frequency for Q (MHz)"=w401:dbl)  [unwired: 1 out]
            n203 = call "WS1021 demo read error limits.vi"("file path (dialog if empty)"=w390) -> ("Error limits"=→"Error limits":cluster{"Array":i32[], "Array":dbl[]})  [unwired: 8 in, 2 out]
            n204 = property on="OTP" class="Slide (strict)"("Maximum"=w400, "Scale.Maximum"=w400) -> ()  [unwired: 2 in, 2 out]
            n205 = Format Into String(format string="Capacitance (pF)\n at %#gMHz", w402) -> (resulting string=w407:string, error out=w406:errorcluster)  [unwired: 2 in]
            n206 = Format Into String(format string="Q-Value \nat %#gMHz", w401) -> (resulting string=w408:string, error out=w405:errorcluster)  [unwired: 2 in]
            n207 = property on="Capacitance (pF) at f1" class="DigNum (strict)"(error in=w406, "Caption.Text"=w407) -> ()  [unwired: 1 in, 2 out]
            n208 = property on="Q at f2" class="DigNum (strict)"(error in=w405, "Caption.Text"=w408) -> ()  [unwired: 1 in, 2 out]
          }
          frame "Pause" {
            n209 = property on="Pause Button" class="Bool (strict)"() -> (error out=w411:errorcluster, "Value"=w413:bool)  [unwired: 2 in, 1 out]
            n210 = Not(x=w413) -> (.not. x?=w412:bool)
            n211 = property on="Pause Button" class="Bool (strict)"(error in=w411, "Val(Sgnl)"=w412) -> ()  [unwired: 1 in, 2 out]
          }
        }
      }
    }
    n212 = Get Date/Time String(want seconds? (F)=TRUE) -> (date string=w40:string, time string=w41:string)  [unwired: 2 in]
    n213 = Concatenate Strings(w40, " - " ("string"), w41) -> (→"Time":string)
  }
  "Vector Network Analyzer.lvclass 2" <- w19
  "Error Out" <- w18
  "Toggle 8.lvclass 2" <- w16
